vi "Write Sub Panel MSG.vi"(8 "error in (no error)":errorcluster, 10 "Sub Panel MSG":refnum<vi>, 11 "MENSAJE in":refnum<class "MENSAJE.lvclass">) -> (0 "error out":errorcluster, 3 "MENSAJE out":refnum<class "MENSAJE.lvclass">)   [LabVIEW 2020, in "MENSAJE.lvlib" / "MENSAJE.lvclass"]
uses:
  MENSAJE.lvclass
  MENSAJE.lvclass/MENSAJE.ctl
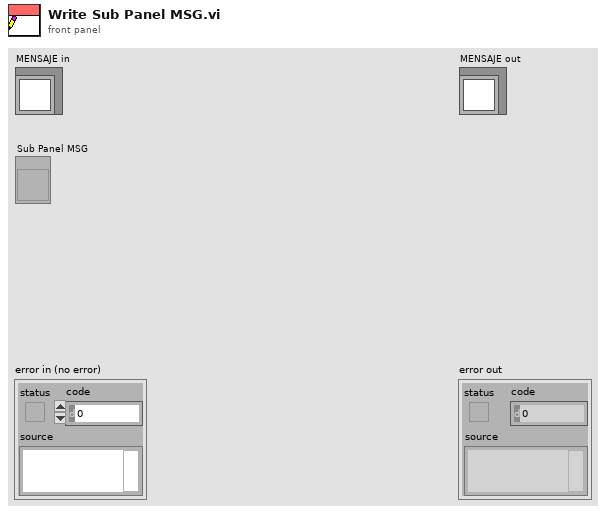
[diagram p1: front panel]
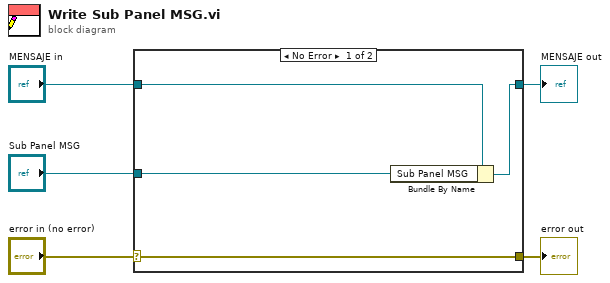
[diagram p0: block diagram]
diagram:
  n1 = case shown="No Error" "error in (no error)" {
    selector: "error in (no error)" -> [w9 w10]
    tunnel: [w9 w10] -> w4
    tunnel: [w7 w11] -> w2
    tunnel: "MENSAJE in" -> [w8 w11]
    tunnel: "Sub Panel MSG" -> [w6 _]
    frame No Error {
      n2 = Bundle By Name(cluster=w8, "Sub Panel MSG"=w6) -> (w7:refnum<class "MENSAJE.lvclass">)
    }
    frame Error {
    }
  }
  "error out" <- w4
  "MENSAJE out" <- w2
